vi "Filter and Sort Items.vi"(5 "Sort Info":T1={"Sort Column"=enum."Description", "Ascending?"=FALSE, "Enabled?"=FALSE}, 7 "Filter Info":T3={"Filter Column"=enum."Description", "Filter Type"=enum."Contains", "Filter Value"="", "New Data?"=FALSE, "Case Sensitive?"=FALSE, "Enabled?"=FALSE}, 8 "error in (no error)":errorcluster, 10 "New Item Data":refnum<class "Item.lvclass">[](array[class]), 11 "Saved Item Data":refnum<class "Item.lvclass">[](array[class])) -> (0 "error out":errorcluster, 1 "Displayed Indices":i32[](array[numeric]), 2 "New Item Data out":refnum<class "Item.lvclass">[](array[class]), 3 "Saved Item Data out":refnum<class "Item.lvclass">[](array[class]))   [LabVIEW 2020, in "VI Properties Editor.lvlib"]
doc: "Filters and sorts either <B>Saved Item Data</B> or <B>New Item Data</B> according to <B>Filter Info</B> and <B>Sort Info</B>."
uses:
  VI Properties Editor.lvlib
  Classes/Item/Item.lvclass
  CTLs/Filter Info.ctl
  CTLs/Filter Column.ctl
  CTLs/Filter Type.ctl
  CTLs/Sort Info.ctl
  CTLs/Sort Column.ctl
  30de6eac-96d7-4eca-b57b-80e4eae92856.vi
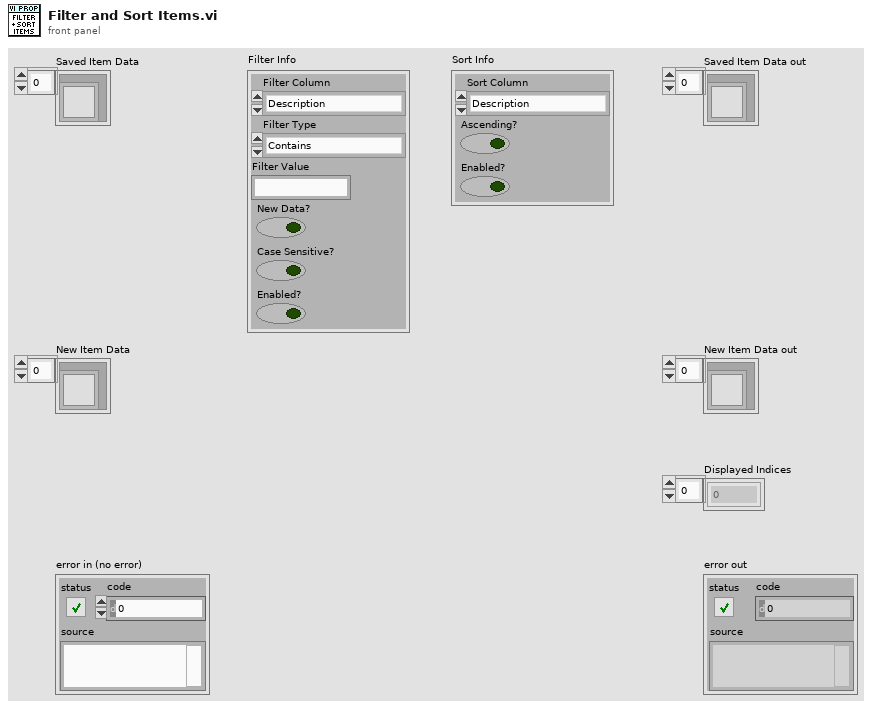
[diagram p1: front panel]
types:
  T1 = typedef "VI Properties Editor.lvlib/Sort Info.ctl" = cluster{"Sort Column":T2, "Ascending?":bool, "Enabled?":bool}
  T2 = typedef "VI Properties Editor.lvlib/Sort Column.ctl" = enum16{"Name", "Filename", "Path", "Type", "Window Title", "Description", "Help Path", "Help Tag", "Custom Title?", "Reentrancy", "Inlined?", "Help URL", "Help Type", "Allow Debugging?", "Auto Error Handling?", "Run When Opened?", "Suspend When Called?", "Priority", "Preferred Exec Sytem"}
  T3 = typedef "VI Properties Editor.lvlib/Filter Info.ctl" = cluster{"Filter Column":T4, "Filter Type":T5, "Filter Value":string, "New Data?":bool, "Case Sensitive?":bool, "Enabled?":bool}
  T4 = typedef "VI Properties Editor.lvlib/Filter Column.ctl" = enum16{"Name", "Path", "Type", "Window Title", "Description", "Help Path", "Help Tag", "Custom Title?", "Reentrancy", "Inlined?", "Help URL", "Help Type", "Allow Debugging?", "Auto Error Handling?", "Run When Opened?", "Suspend When Called?", "Priority", "Preferred Exec Sytem", "Control Label", "Control Caption", "Control Description", "Control Tip Strip"}
  T5 = typedef "VI Properties Editor.lvlib/Filter Type.ctl" = enum16{"Contains", "Equals", "Starts with", "Ends with", "Is empty", "Does not contain", "Does not equal", "Is not empty"}
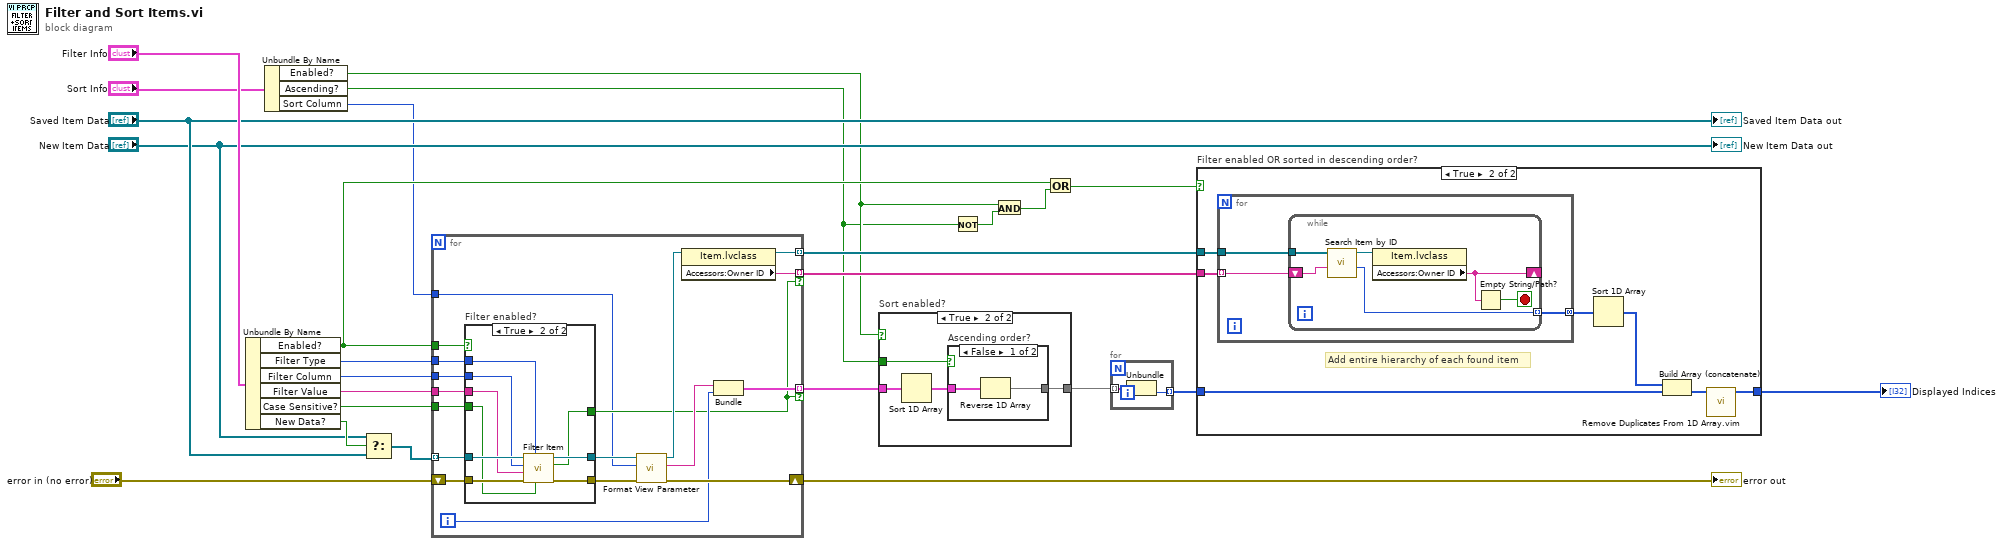
[diagram p0: block diagram]
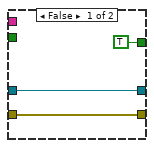
[diagram p2: hidden frame]
diagram:
  n1 = Unbundle By Name("Filter Info") -> ("Enabled?"=w16:bool, "Filter Type"=w22:T5, "Filter Column"=w14:T4, "Filter Value"=w15:string, "Case Sensitive?"=w1:bool, "New Data?"=w18:bool)
  n2 = Unbundle By Name("Sort Info") -> ("Enabled?"=w4:bool, "Ascending?"=w3:bool, "Sort Column"=w13:T2)
  n3 = Select(t="New Item Data", s=w18, f="Saved Item Data") -> (s? t:f=w19:refnum<class "Item.lvclass">[])
  n4 = for {
    tunnel: w19 -> [w38] mode=indexing
    tunnel: w14 -> [w37]
    tunnel: w22 -> [w32]
    tunnel: w15 -> [w33]
    tunnel: [w40] -> w12 mode=indexing if=w28
    tunnel: w13 -> [w27]
    shift-right: [w41] -> w24
    shift-left: "error in (no error)" -> [w43]
    tunnel: [w36] -> w11 mode=indexing if=w28
    tunnel: [w35] -> w10 mode=indexing
    tunnel: w16 -> [w30]
    tunnel: w1 -> [w26]
    i -> [w34]
    n5 = case "Filter enabled?" shown="True" w30 {
      tunnel: w38 -> [w45 w53]
      tunnel: w37 -> [_ w52]
      tunnel: w43 -> [w46 w55]
      tunnel: w33 -> [_ w51]
      tunnel: w32 -> [_ w50]
      tunnel: [w46 w54] -> w42
      tunnel: [w45 w49] -> w31
      tunnel: [TRUE ("Include?") w48] -> w28
      tunnel: w26 -> [_ w47]
      frame False {
      }
      frame True {
        n6 = call-dynamic "Filter Item.vi"("Case Sensitive?"=w47, "Filter Type"=w50, "error in (no error)"=w55, "Filter Value"=w51, "Filter Column"=w52, "Item in"=w53) -> ("error out"=w54:errorcluster, "Include?"=w48:bool, "Item out"=w49:refnum<class "Item.lvclass">)  [unwired: 3 in]
      }
    }
    n7 = call-dynamic "Format View Parameter.vi"("error in (no error)"=w42, "Column"=w27, "Item in"=w31) -> ("error out"=w41:errorcluster, "View Parameter"=w39:string, "Item out"=w29:refnum<class "Item.lvclass">)  [unwired: 6 in]
    n8 = property class="Item.lvclass"(reference=w29) -> (reference out=w35:refnum<class "Item.lvclass">, "Accessors:Owner ID"=w36:string)  [unwired: 1 in, 1 out]
    n9 = Bundle("View Parameter"=w39, w34) -> (w40:cluster{"View Parameter":string, i32})  [unwired: 1 in]
  }
  "error out" <- w24
  n10 = case "Sort enabled?" shown="True" w4 {
    tunnel: w12 -> [w56 w60]
    tunnel: [w56 w58] -> w8
    tunnel: w3 -> [_ w57]
    frame False {
    }
    frame True {
      n11 = Sort 1D Array(array=w60) -> (sorted array=w59:cluster{"View Parameter":string, i32}[])
      n12 = case "Ascending order?" shown="False" w57 {
        tunnel: w59 -> [w62 w63]
        tunnel: [w61 w63] -> w58
        frame False {
          n13 = Reverse 1D Array(array=w62) -> (reversed array=w61:cluster{"View Parameter":string, i32}[])
        }
        frame True {
        }
      }
    }
  }
  n14 = Not(x=w3) -> (.not. x?=w5:bool)
  n15 = And(x=w4, y=w5) -> (x .and. y?=w2:bool)
  n16 = Or(x=w16, y=w2) -> (x .or. y?=w6:bool)
  n17 = for {
    tunnel: w8 -> [w65] mode=indexing
    tunnel: [w64] -> w9 mode=indexing
    n18 = Unbundle(w65) -> (w64:i32)  [unwired: 1 out]
  }
  n19 = case "Filter enabled OR sorted in descending order?" shown="True" w6 {
    tunnel: w11 -> [_ w73]
    tunnel: w10 -> [_ w72]
    tunnel: w9 -> [w66 w71]
    tunnel: [w66 w67] -> w7
    frame False {
    }
    frame True {
      # "Add entire hierarchy of each found item"
      n20 = for {
        tunnel: w73 -> [w75] mode=indexing
        tunnel: w72 -> [w76]
        tunnel: [w74] -> w69 mode=concatenating
        n21 = while {
          tunnel: w76 -> [w82]
          shift-right: [w78] -> _
          shift-left: w75 -> [w81]
          tunnel: [w77] -> w74 mode=indexing
          stop <- w79 stop-if-true
          n22 = call "Search Item by ID.vi"("Item ID"=w81, "Items"=w82) -> ("Index"=w77:i32, "Item"=w80:refnum<class "Item.lvclass">)  [unwired: 8 in]
          n23 = property class="Item.lvclass"(reference=w80) -> ("Accessors:Owner ID"=w78:string)  [unwired: 1 in, 2 out]
          n24 = Empty String/Path?(string/path=w78) -> (empty?=w79:bool)
        }
      }
      n25 = Sort 1D Array(array=w69) -> (sorted array=w68:i32[])
      n26 = Build Array (concatenate)(w68, w71) -> (w70:i32[])
      n27 = call "Remove Duplicates From 1D Array.vim"("array"=w70) -> ("array with duplicates removed"=w67:i32[])  [unwired: 10 in]
    }
  }
  "Displayed Indices" <- w7
  "Saved Item Data out" <- "Saved Item Data"
  "New Item Data out" <- "New Item Data"
